vi "NUC.vi"(0 "image in":refnum<class "MSC Image.lvclass">, 1 "NUC Table":T1, 5 "error in (no error)":errorcluster) -> (14 "image out":refnum<class "MSC Image.lvclass">, 19 "error out":errorcluster)   [LabVIEW 2016, in "MSC Image.lvclass"]
doc: "After the estimation of the NUC table is done, it is possible to apply the correction on an image.\n\nFor more information about this process please check the documentation."
uses:
  MSC Image.lvclass
  controls/Image Type.ctl
  controls/NUC Table.ctl
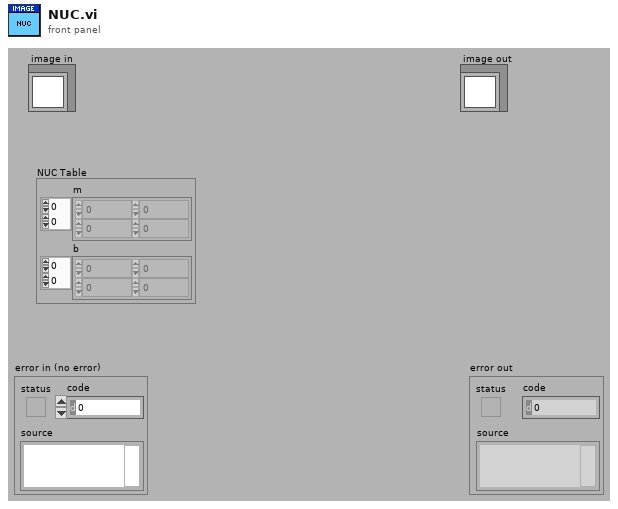
[diagram p1: front panel]
types:
  T1 = typedef "MSC Image.lvclass/NUC Table.ctl" = cluster{"m":dbl[][], "b":dbl[][]}
  T2 = typedef "MSC Image.lvclass/Image Type.ctl" = i32
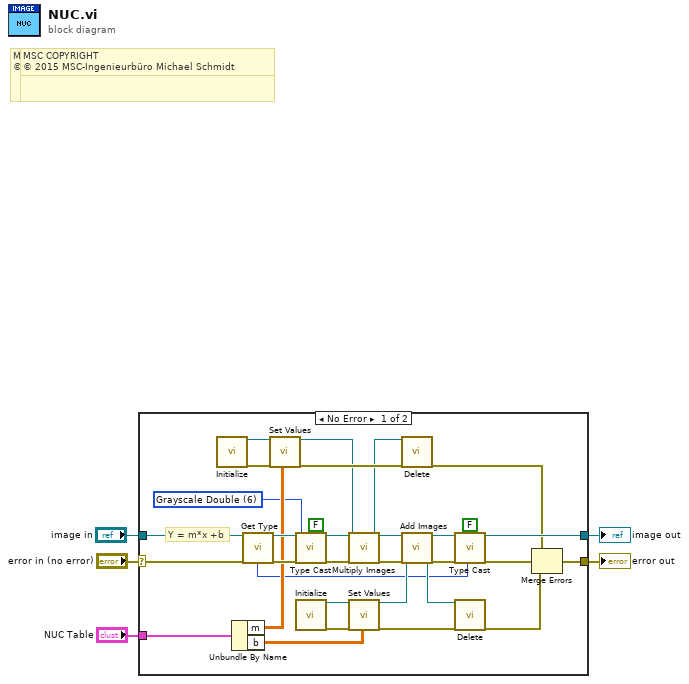
[diagram p0: block diagram]
diagram:
  # "MSC COPYRIGHT\n© 2016 MSC-Ingenieurbüro Michael Schmidt"
  # "MSC COPYRIGHT\n© 2016 MSC-Ingenieurbüro Michael Schmidt"
  # "MSC COPYRIGHT\n© 2015 MSC-Ingenieurbüro Michael Schmidt"
  # "MSC COPYRIGHT\n© 2015 MSC-Ingenieurbüro Michael Schmidt"
  n1 = case shown="No Error" "error in (no error)" {
    selector: "error in (no error)" -> [w23 w39]
    tunnel: [w14 w39] -> w4
    tunnel: [w25 w38] -> w2
    tunnel: "image in" -> [w29 w38]
    tunnel: "NUC Table" -> [w24 _]
    frame No Error {
      w7 = T2 6 items=["Grayscale U8"=0, "Grayscale U16"=2, "Grayscale Single"=5, "Grayscale Double"=6, "RGB U8"=16] ("Image Type")
      # "Y = m*x +b"
      n2 = call "Initialize.vi"() -> ("image out"=w35:refnum<class "MSC Image.lvclass">, "error out"=w34:errorcluster)  [unwired: 18 in]
      n3 = Unbundle By Name(w24) -> ("m"=w11:dbl[][], "b"=w10:dbl[][])
      n4 = call-dynamic "Get Type.vi"("image in"=w29, "error in (no error)"=w23) -> ("image out"=w28:refnum<class "MSC Image.lvclass">, "Image Type"=w6:T2, "error out"=w22:errorcluster)  [unwired: 15 in]
      n5 = call-dynamic "Set Values.vi"("image in"=w35, "imageData Double"=w11, "error in (no error)"=w34) -> ("image out"=w9:refnum<class "MSC Image.lvclass">, "error out"=w19:errorcluster)  [unwired: 15 in]
      n6 = call-dynamic "Type Cast.vi"("image in"=w28, "Image Type"=w7, "Scale?"=FALSE, "error in (no error)"=w22) -> ("image out"=w27:refnum<class "MSC Image.lvclass">, "error out"=w21:errorcluster)  [unwired: 14 in]
      n7 = call "Initialize.vi"() -> ("image out"=w37:refnum<class "MSC Image.lvclass">, "error out"=w36:errorcluster)  [unwired: 18 in]
      n8 = call-dynamic "Multiply Images.vi"("image in"=w27, "image 2 in"=w9, "error in (no error)"=w21) -> ("image out"=w26:refnum<class "MSC Image.lvclass">, "image 2 out"=w8:refnum<class "MSC Image.lvclass">, "error out"=w20:errorcluster)  [unwired: 14 in]
      n9 = call-dynamic "Set Values.vi"("image in"=w37, "imageData Double"=w10, "error in (no error)"=w36) -> ("image out"=w13:refnum<class "MSC Image.lvclass">, "error out"=w18:errorcluster)  [unwired: 15 in]
      n10 = call-dynamic "Delete.vi"("image in"=w8, "error in (no error)"=w19) -> ("error out"=w15:errorcluster)  [unwired: 17 in]
      n11 = call-dynamic "Add Images.vi"("image in"=w26, "image 2 in"=w13, "error in (no error)"=w20) -> ("image out"=w33:refnum<class "MSC Image.lvclass">, "image 2 out"=w12:refnum<class "MSC Image.lvclass">, "error out"=w32:errorcluster)  [unwired: 14 in]
      n12 = call-dynamic "Type Cast.vi"("image in"=w33, "Image Type"=w6, "Scale?"=FALSE, "error in (no error)"=w32) -> ("image out"=w25:refnum<class "MSC Image.lvclass">, "error out"=w16:errorcluster)  [unwired: 14 in]
      n13 = call-dynamic "Delete.vi"("image in"=w12, "error in (no error)"=w18) -> ("error out"=w17:errorcluster)  [unwired: 17 in]
      n14 = Merge Errors(w15, w16, w17) -> (w14:errorcluster)
    }
    frame Error {
    }
  }
  "error out" <- w4
  "image out" <- w2
